vi "保存数据.vi"(11 "数组":string[][](array[string])) -> ()   [LabVIEW 2018, in "qingshan.lvlib"]
uses:
  qingshan/qingshan.lvlib
panel:
  out "character string":string caption="字符串"
  out "长度":i32
  out "文本":string
  in  "错误输入":errorcluster
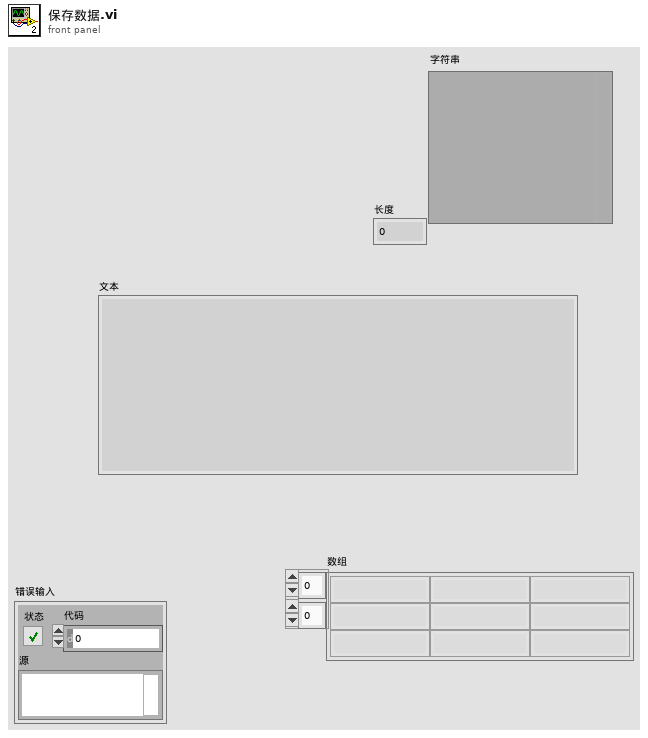
[diagram p1: front panel]
types:
  T1 = enum16{"open", "replace", "create", "open or create", "replace or create", "replace or create with confirmation"}
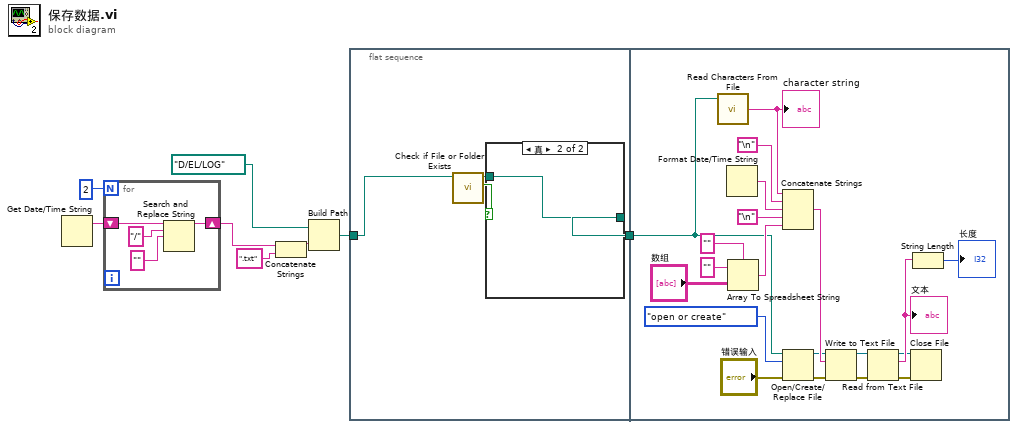
[diagram p0: block diagram]
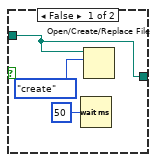
[diagram p2: hidden frame]
diagram:
  n1 = Get Date/Time String() -> (date string=w6:string)  [unwired: 3 in, 1 out]
  n2 = for {
    N: 2 -> [_]
    shift-right: [w10] -> w4
    shift-left: w6 -> [w12]
    n3 = Search and Replace String(input string=w12, search string="/" ("搜索字符串"), replace string="" ("替换字符串(\"\")")) -> (result string=w10:string)  [unwired: 5 in, 3 out]
  }
  n4 = Concatenate Strings(w4, ".txt" ("字符串")) -> (w7:string)
  n5 = Build Path(base path=path "D:/EL/LOG" ("基路径"), name or relative path=w7) -> (appended path=w3:path)
  n6 = flat-sequence {
    tunnel: w3 -> [w16]
    tunnel: [w14] -> w2
    tunnel: w2 -> [w23]
    frame #0 {
      n7 = call <vilib>:"Check if File or Folder Exists.vi"("path"=w16) -> ("file or folder exists?"=w15:bool, "dup path"=w13:path)  [unwired: 8 in, 1 out]
      n8 = case shown="真" w15 {
        tunnel: [w18 w20] -> w14
        tunnel: w13 -> [w18 w20]
        frame False {
          n9 = Wait (ms)(milliseconds to wait=u32 50 ("等待时间（毫秒）")) -> ()  [unwired: 1 out]
          n10 = Open/Create/Replace File(file path (use dialog)=w18, operation (0:open)=T1."create" ("操作(0:open)")) -> ()  [unwired: 4 in, 3 out]
        }
        frame True {
        }
      }
    }
    frame #1 {
      n11 = call <vilib>:"Read Characters From File.vi"("file path (dialog if empty)"=w23) -> ("character string"=w25:string)  [unwired: 5 in, 3 out]
      "character string" <- w25
      n12 = Format Date/Time String() -> (date/time string=w37:string)  [unwired: 3 in]
      n13 = Array To Spreadsheet String ("数组至电子表格字符串转换")(delimiter (Tab)="" ("分隔符(Tab)"), array="数组", 3:"" ("格式字符串")) -> (spreadsheet string=w32:string)
      n14 = Concatenate Strings(w25, "\n", w37, "\n", w32) -> (w35:string)
      n15 = Open/Create/Replace File ("打开/创建/替换文件")(file path (use dialog)=w23, error in="错误输入", operation (0:open)=T1."open or create" ("操作(0:open)")) -> (refnum out=w22:refnum<file>, error out=w21:errorcluster)  [unwired: 3 in, 1 out]
      n16 = Write to Text File ("写入文本文件")(file (use dialog)=w22, text=w35, error in=w21) -> (refnum out=w30:refnum<file>, error out=w31:errorcluster)  [unwired: 1 in, 1 out]
      n17 = Read from Text File ("读取文本文件")(file (use dialog)=w30, error in=w31) -> (refnum out=w27:refnum<file>, text=w28:string, error out=w26:errorcluster)  [unwired: 2 in, 1 out]
      "文本" <- w28
      n18 = Close File(refnum=w27, error in=w26) -> ()  [unwired: 2 out]
      n19 = String Length(string=w28) -> (length=→"长度":i32)
    }
  }
